vi "Read Stepper Configuration.vi"(8 "error in (no error)":errorcluster, 11 "Stepper in":refnum<class "Stepper.lvclass">) -> (0 "error out":errorcluster, 2 "Stepper Configuration":T1={"Start"=-0.001, "End"=0.001, "Step"=0.0001, "Append measurements"=[]} {"Step" format="%#_6p"; "End" format="%#_6p"; "Start" format="%#_6p"}, 3 "Stepper out":refnum<class "Stepper.lvclass">)   [LabVIEW 2021, in "Stepper.lvclass"]
uses:
  Stepper.lvclass
  Stepper.lvclass/Stepper.ctl
  NHMFL_Core/Libraries/Instruments/Controls/Stepper Config.ctl
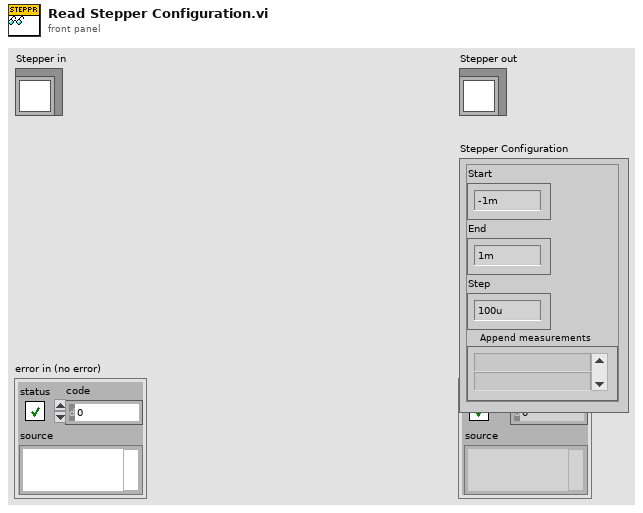
[diagram p1: front panel]
types:
  T1 = typedef "Stepper Config.ctl" = cluster{"Start":dbl, "End":dbl, "Step":dbl, "Append measurements":string[]}
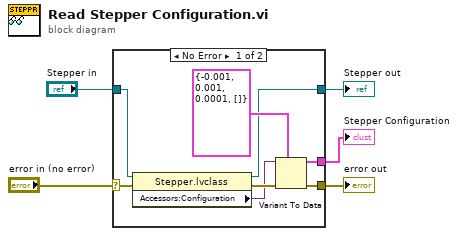
[diagram p0: block diagram]
diagram:
  n1 = case shown="No Error" "error in (no error)" {
    selector: "error in (no error)" -> [w13 w14]
    tunnel: [w12 w14] -> w4
    tunnel: [w8 w15] -> w2
    tunnel: "Stepper in" -> [w9 w15]
    tunnel: [w6 _] -> w1
    frame No Error {
      n2 = property class="Stepper.lvclass"(reference=w9, error in=w13) -> (reference out=w8:refnum<class "Stepper.lvclass">, error out=w10:errorcluster, "Accessors:Configuration"=w7:variant)
      n3 = Variant To Data(error in=w10, type=T1 {"Start"=-0.001, "End"=0.001, "Step"=0.0001, "Append measurements"=[]} ("Configuration"), Variant=w7) -> (data=w6:T1, error out=w12:errorcluster)
    }
    frame Error {
    }
  }
  "error out" <- w4
  "Stepper out" <- w2
  "Stepper Configuration" <- w1
